vi "ExSubNframeColMultiImageFastDPH.vi"(1 "image handles":u32[](array[numeric]), 3 "error in (no error)":errorcluster, 4 "Number of Images":u32=1 min=1 step=1, 6 "Handle Cluster":T1) -> (0 "error out":errorcluster, 2 "Handle Cluster":T1, 5 "data handles":u32[](array[numeric]))   [LabVIEW 2012]
panel:
  # "ExSubNframeCol:\nThis is a sub VI that collects N frames from the camera\nsystem. This assumes camera has been setup and \ninitialized and that the start camera is done. It also \nassumes the camera has circular buffer capabillities.\nThis is not true for all cameras, especially older \nPhotometrics cameras."
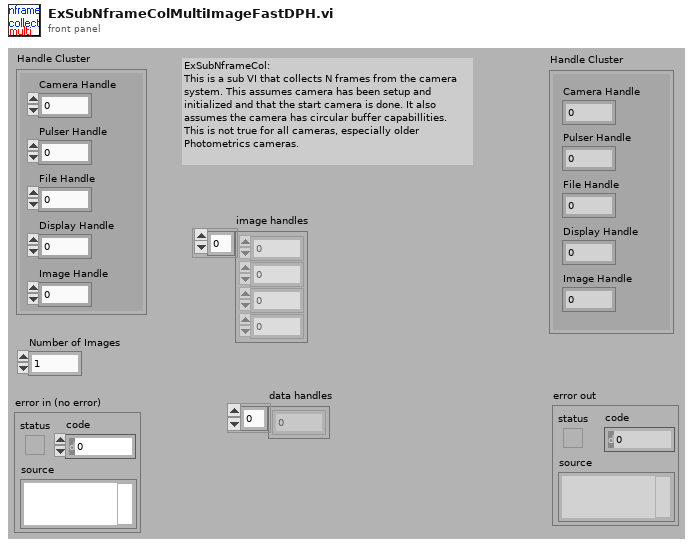
[diagram p1: front panel]
types:
  T1 = cluster{"Camera Handle":u32, "Pulser Handle":u32, "File Handle":u32, "Display Handle":u32, "Image Handle":u32}
  T2 = cluster{"Camera Handle":u32, "Pulser Handle":u32, "File Handle":u32, "Display Handle":u32, "Data Handle":u32}
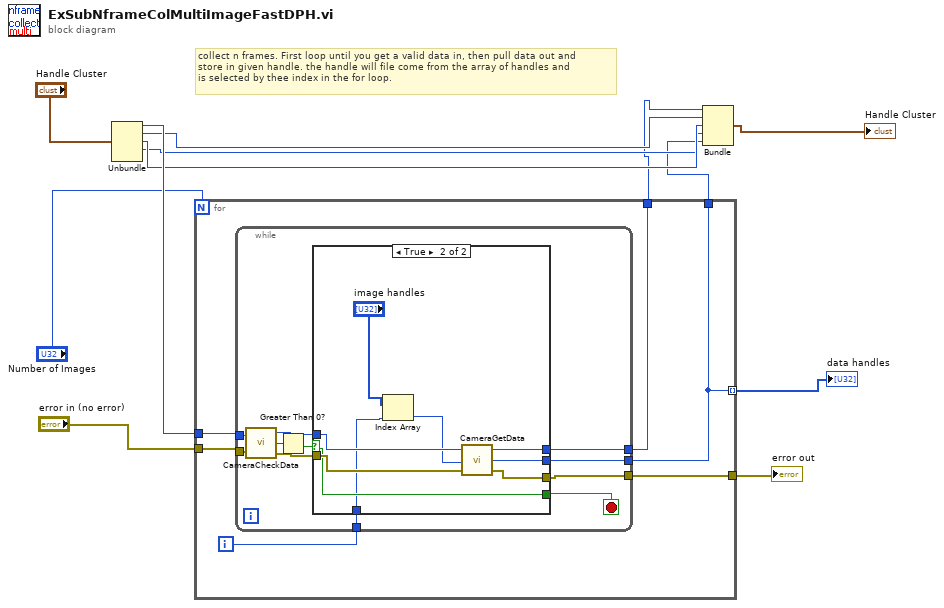
[diagram p0: block diagram]
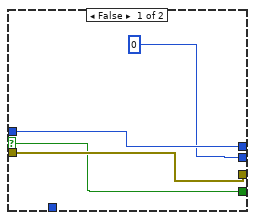
[diagram p2: hidden frame]
diagram:
  # "collect n frames. First loop until you get a valid data in, then pull data out and \nstore in given handle. the handle will file come from the array of handles and\nis selected by thee index in the for loop."
  n1 = Unbundle("Handle Cluster") -> ("Camera Handle"=w12:u32, "Pulser Handle"=w7:u32, "File Handle"=w6:u32, "Display Handle"=w5:u32)  [unwired: 1 out]
  n2 = for {
    N: "Number of Images" -> [_]
    tunnel: w12 -> [w18]
    tunnel: "error in (no error)" -> [w17]
    tunnel: [w15] -> w8
    tunnel: [w14] -> w1
    tunnel: [w13] -> w4
    tunnel: [w13] -> w2 mode=indexing
    i -> [w16]
    n3 = while {
      tunnel: w17 -> [w28]
      tunnel: w18 -> [w27]
      tunnel: [w22] -> w15
      tunnel: w16 -> [w21]
      tunnel: [w20] -> w14
      tunnel: [w19] -> w13
      stop <- w23 stop-if-true
      n4 = call <userlib>:"CameraCheckData.vi"("Camera Handle"=w27, "error in"=w28) -> ("Camera Handle"=w25:u32, "Number Of Frames Available"=w29:i32, "error out"=w24:errorcluster)
      n5 = Greater Than 0?(x=w29) -> (x > 0?=w26:bool)
      n6 = case shown="True" w26 {
        selector: w26 -> [w32 w40]
        tunnel: w25 -> [w31 w42]
        tunnel: w24 -> [w33 w41]
        tunnel: [w32 w40] -> w23
        tunnel: [w33 w36] -> w22
        tunnel: w21 -> [_ w39]
        tunnel: [w31 w35] -> w20
        tunnel: [0 w34] -> w19
        frame False {
        }
        frame True {
          n7 = Index Array(array="image handles", index=w39) -> (element=w37:u32)
          n8 = call <userlib>:"CameraGetData.vi"("error in"=w41, "Data Handle"=w37, "Camera Handle"=w42) -> ("error out"=w36:errorcluster, "Data Handle"=w34:u32, "Camera Handle"=w35:u32)
        }
      }
    }
  }
  "error out" <- w8
  "data handles" <- w2
  n9 = Bundle("Camera Handle"=w1, "Pulser Handle"=w7, "File Handle"=w6, "Display Handle"=w5, "Data Handle"=w4) -> (→"Handle Cluster":T2)  [unwired: 1 in]
